vi "Query Motor Position (TRIAX).vi"(7 "Mono System # (0)":T1, 8 "error in (no error)":errorcluster, 11 "VISA resource name":refnum<visa-resource-name>) -> (0 "error out":errorcluster, 2 "wavelength":dbl[unit], 3 "VISA resource name out":refnum<visa-resource-name>)   [LabVIEW 2009, in "JY-SPEX-TRIAX.lvlib"]
doc: "Queries the current wavelength setting according to the base grating (1200 grooves/mm).\n\n<B>Note: only works with TRIAX series monochromators.</B>"
uses:
  JY-SPEX-TRIAX.lvlib
  controls.llb/Monochromator System Number.ctl
  Spectrometer Config.vi
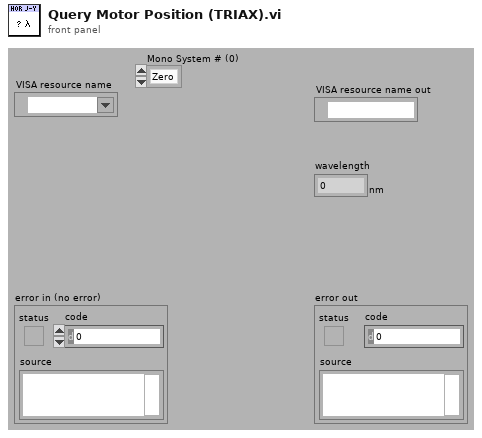
[diagram p1: front panel]
types:
  T1 = typedef "JY-SPEX-TRIAX.lvlib/Monochromator System Number.ctl" = enum16{"Zero", "One"}
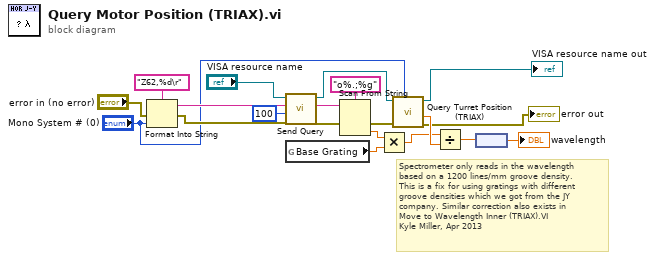
[diagram p0: block diagram]
diagram:
  # "Spectrometer only reads in the wavelength\nbased on a 1200 lines/mm groove density.\nThis is a fix for using gratings with different\ngroove densities which we got from the JY\ncompany. Similar correction also exists in \nMove to Wavelength Inner (TRIAX).VI\nKyle Miller, Apr 2013"
  n1 = Format Into String(format string="Z62,%d\r", error in="error in (no error)", "Mono System # (0)") -> (resulting string=w13:string, error out=w11:errorcluster)  [unwired: 1 in]
  n2 = call "Send Query.vi"("error in (no error)"=w11, "byte count"=u32 100, "write buffer"=w13, "VISA resource name"="VISA resource name") -> ("error out"=w16:errorcluster, "read buffer"=w18:string, "VISA resource name out"=w10:refnum<visa-resource-name>)  [unwired: 5 out]
  n3 = global read "Spectrometer Config.vi" "Base Grating"() -> (w8:dbl[unit])
  n4 = Scan From String(format string="o%.;%g", input string=w18, error in=w16) -> (error out=w2:errorcluster, output 1=w9:dbl)  [unwired: 1 in, 3 out]
  n5 = Multiply(x=w9, y=w8) -> (x*y=w6:dbl[unit])
  n6 = call "Query Turret Position (TRIAX).vi"("Mono System # (0)"="Mono System # (0)", "error in (no error)"=w2, "VISA resource name"=w10) -> ("error out"=→"error out":errorcluster, "Groove Density"=w7:dbl[unit], "VISA resource name out"=→"VISA resource name out":refnum<visa-resource-name>)  [unwired: 4 in, 2 out]
  n7 = Divide(x=w6, y=w7) -> (x/y=w5:dbl)
  n8 = node(w5) -> (→"wavelength":dbl[unit])
